vi "Follow.vi"() -> ()   [LabVIEW 2014]
panel:
  in  "stop":bool
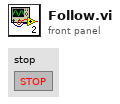
[diagram p1: front panel]
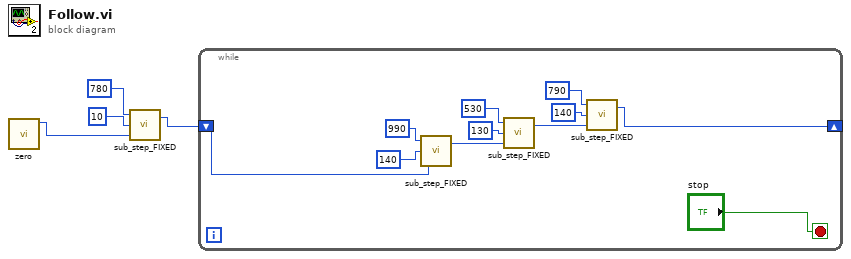
[diagram p0: block diagram]
diagram:
  n1 = call "zero.vi"() -> ("PositionOut"=w2:i32)  [unwired: 11 in]
  n2 = call "sub_step_FIXED.vi"("Current Position"=w2, "millisecond multiple"=u32 10, "Desired Position"=780) -> ("Position Out"=w1:i32)  [unwired: 1 in]
  n3 = while {
    shift-right: [w5] -> _
    shift-left: w1 -> [w6]
    stop <- "stop" stop-if-true
    n4 = call "sub_step_FIXED.vi"("Current Position"=w6, "millisecond multiple"=u32 140, "Desired Position"=990) -> ("Position Out"=w10:i32)  [unwired: 1 in]
    n5 = call "sub_step_FIXED.vi"("Current Position"=w10, "millisecond multiple"=u32 130, "Desired Position"=530) -> ("Position Out"=w9:i32)  [unwired: 1 in]
    n6 = call "sub_step_FIXED.vi"("Current Position"=w9, "millisecond multiple"=u32 140, "Desired Position"=790) -> ("Position Out"=w5:i32)  [unwired: 1 in]
  }
